vi "LeCroy.Read Scan Histo.vi"(8 "Error In":errorcluster, 11 "LeCroy.Session in":T1) -> (0 "Error Out":errorcluster, 2 "waveform":waveform(dbl), 3 "LeCroy.Session out":T1)   [LabVIEW 2018]
uses:
  typedefs/LeCroy.Session.ctl
  Driver/lecroy_wave_series/LeCroy Wave Series/Public/Data/Read Single Raw Waveform.vi
  Driver/lecroy_wave_series/LeCroy Wave Series/LeCroy Wave Series.lvlib
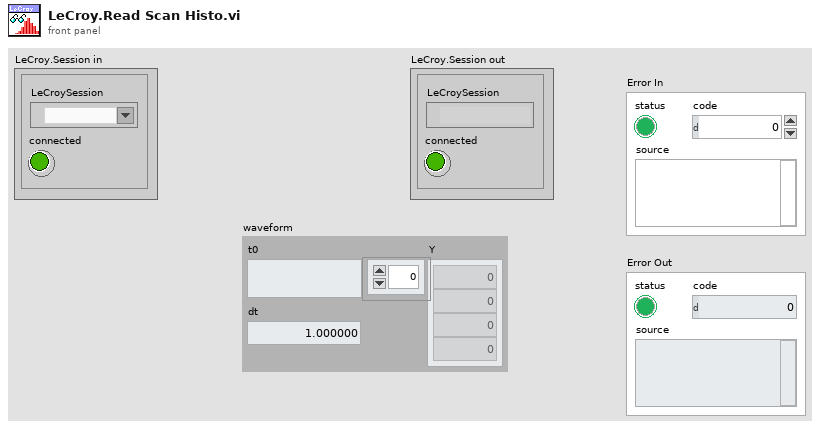
[diagram p1: front panel]
types:
  T1 = typedef "LeCroy.Session.ctl" = cluster{"LeCroySession":refnum<visa-resource-name>, "connected":bool}
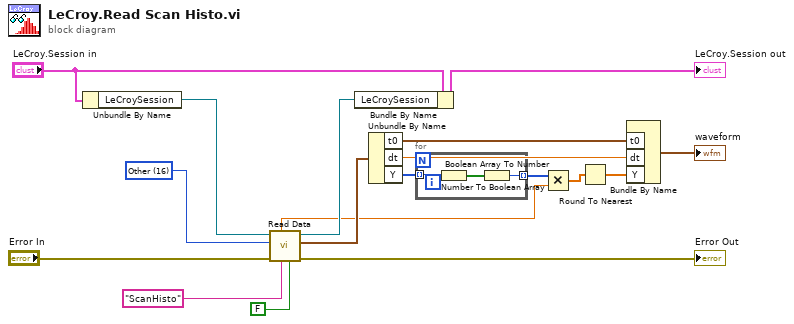
[diagram p0: block diagram]
diagram:
  w12 = u16 16 items=["Channel 1", "Channel 2", "Channel 3", "Channel 4", "Memory 1", "Memory 2", "Memory 3", "Memory 4", "Function 1", "Function 2", "Function 3", "Function 4", "Function 5", "Function 6", "Function 7", "Function 8", "Other"] ("Source (0: Channel 1)")
  n1 = Unbundle By Name("LeCroy.Session in") -> ("LeCroySession"=w16:refnum<visa-resource-name>)
  n2 = call-poly "Read Data.vi"("Arm trigger"=FALSE, "Custom Source ID"="ScanHisto", "error in (no error)"="Error In", "Source (0: Channel 1)"=w12, "VISA resource name"=w16) -> ("error out"=→"Error Out":errorcluster, "Waveform Data"=w9:waveform(i16), "VISA resource name out"=w15:refnum<visa-resource-name>, "Vertical gain"=w3:sgl)  [unwired: 2 in, 1 out]
  n3 = Bundle By Name(cluster="LeCroy.Session in", "LeCroySession"=w15) -> (→"LeCroy.Session out":T1)
  n4 = Unbundle By Name(w9) -> ("t0"=w6:timestamp, "dt"=w7:dbl, "Y"=w4:i16[])
  n5 = for {
    tunnel: w4 -> [w21] mode=indexing
    tunnel: [w19] -> w2 mode=indexing
    n6 = Number To Boolean Array(number=w21) -> (Boolean array=w20:bool[])
    n7 = Boolean Array To Number(Boolean array=w20) -> (number=w19:u32)
  }
  n8 = Multiply(x=w2, y=w3) -> (x*y=w10:sgl[])
  n9 = Round To Nearest(number=w10) -> (nearest integer value=w5:sgl[])
  n10 = Bundle By Name("t0"=w6, "dt"=w7, "Y"=w5) -> (→"waveform":waveform(sgl))  [unwired: 1 in]
